vi "BPM FPGA Filter.vi"(9 "filter?":bool, 11 "input":fxp<+/-,20,5>[](array[numeric])=[0.0, 0.0, 0.0, 0.0, 0.0, 0.0, 0.0, 0.0, 0.0, 0.0]) -> (2 "Internal":fxp<+/-,20,5>[](array[numeric]), 3 "output":fxp<+/-,20,5>[](array[numeric]))   [LabVIEW 2011]
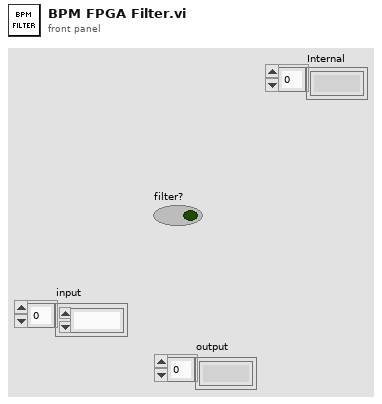
[diagram p1: front panel]
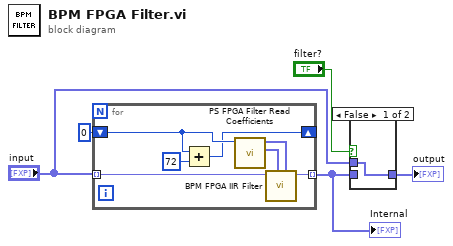
[diagram p0: block diagram]
diagram:
  n1 = for {
    tunnel: "input" -> [w12] mode=indexing
    tunnel: [w11] -> w3 mode=indexing
    shift-right: [w7] -> _
    shift-left: u16 0 -> [w8]
    n2 = Add(x=w8, y=u16 72 ("Number of \nCoefficients\nper Channel")) -> (x+y=w7:u16)
    n3 = call "PS FPGA Filter Read Coefficients.vi"("offset"=w8) -> ("a coeffs"=w9:fxp<+/-,22,4>[], "b coeffs"=w10:fxp<+/-,22,4>[])  [unwired: 9 in]
    n4 = call "BPM FPGA IIR Filter.vi"("coeff_b"=w10, "coeff_a"=w9, "input data"=w12) -> ("output data"=w11:fxp<+/-,20,5>)  [unwired: 8 in]
  }
  "Internal" <- w3
  n5 = case shown="False" "filter?" {
    tunnel: [w13 w14] -> w4
    tunnel: w3 -> [_ w14]
    tunnel: "input" -> [w13 _]
    frame False {
    }
    frame True {
    }
  }
  "output" <- w4
